vi "Get All Default Shortcuts.vi"() -> (0 "All Default Shortcuts":string[](array[string]))   [LabVIEW 2021, in "Seq Edit Quick Drop.lvlib"]
uses:
  Seq Edit Quick Drop.lvlib
  Get Modifier.vi
  Settings.vi
  <vilib>/Utility/error.llb/Trim Whitespace.vi
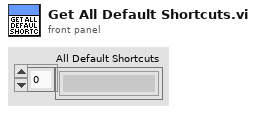
[diagram p1: front panel]
types:
  T1 = cluster{"SHIFT":bool, "CONTROL":bool, "ALT":bool}
  T2 = typedef "Seq Edit Quick Drop.lvlib/Modifiers.ctl" = enum16{"SHIFT", "CTRL", "ALT"}
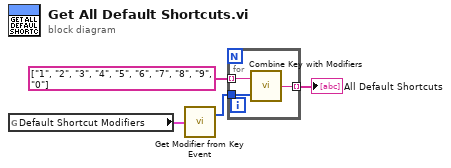
[diagram p0: block diagram]
diagram:
  n1 = global read "Settings.vi" "Default Shortcut Modifiers"() -> (w1:T1)
  n2 = call "Get Modifier from Key Event.vi"("Modifiers"=w1) -> ("Modifiers"=w2:T2[])  [unwired: 1 out]
  n3 = for {
    tunnel: w2 -> [w7]
    tunnel: string[] ["1", "2", "3", "4", "5", "6", "7", "8", "9", "0"] -> [w6] mode=indexing
    tunnel: [w5] -> w4 mode=indexing
    n4 = call "Combine Key with Modifiers.vi"("Modifiers"=w7, "Key"=w6) -> ("Combined"=w5:string)
  }
  "All Default Shortcuts" <- w4
